vi "Set Text Delimiter.vi"(8 "error in (no error)":errorcluster, 10 "Delimiter":string="\t", 11 "Text Log File in":refnum<class "Text Log File.lvclass">) -> (0 "error out":errorcluster, 3 "Text Log File out":refnum<class "Text Log File.lvclass">)   [LabVIEW 2015, in "Waveform Data Logger Engine.lvlib" / "Text Log File.lvclass"]
uses:
  Text Log File.lvclass
  Text Log File.lvclass/Text Log File.ctl
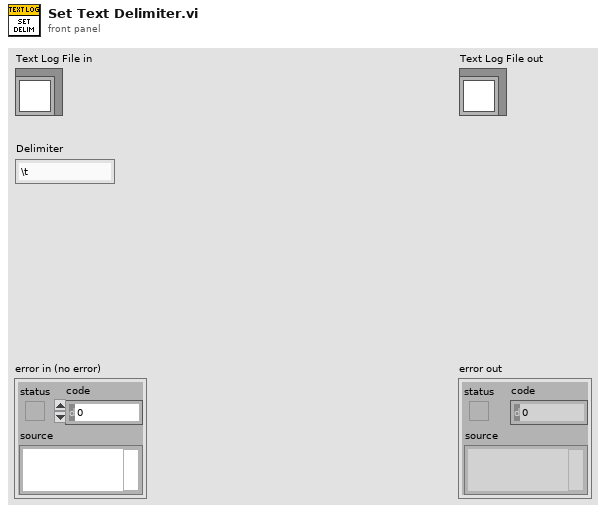
[diagram p1: front panel]
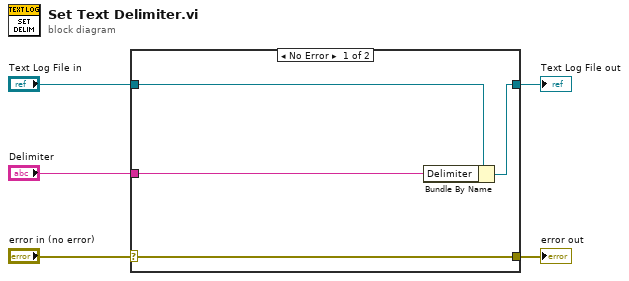
[diagram p0: block diagram]
diagram:
  n1 = case shown="No Error" "error in (no error)" {
    selector: "error in (no error)" -> [w9 w10]
    tunnel: [w9 w10] -> w4
    tunnel: [w7 w11] -> w2
    tunnel: "Text Log File in" -> [w8 w11]
    tunnel: "Delimiter" -> [w6 _]
    frame No Error {
      n2 = Bundle By Name(cluster=w8, "Delimiter"=w6) -> (w7:refnum<class "Text Log File.lvclass">)
    }
    frame Error {
    }
  }
  "error out" <- w4
  "Text Log File out" <- w2
